vi "Do.vi"(8 "error in (no error)":errorcluster, 10 "Actor in":refnum<class "Actor.lvclass">, 11 "Get Indicators":refnum<class "Get Indicators.lvclass">) -> (0 "error out":errorcluster, 2 "Actor out":refnum<class "Actor.lvclass">)   [LabVIEW 2014, in "tWorkerCommandRunner.lvlib" / "Get Indicators.lvclass"]
doc: "(<B>Filename</B>: Actor Framework.lvlib:Message.lvclass:Do.vi)\n\nDefines what a message does when it is received by an actor. Generally, a message instructs an actor to invoke one of its methods. By default, this method does nothing. A child class must override it to define behavior. Create a child class by using the Actor Framework Message Maker dialog box."
uses:
  Get Indicators.lvclass
  <vilib>/ActorFramework/Actor/Actor.lvclass
  tWorkerCommandRunner/tWorkerCommandRunner.lvclass
  Get Indicators.lvclass/Get Indicators.ctl
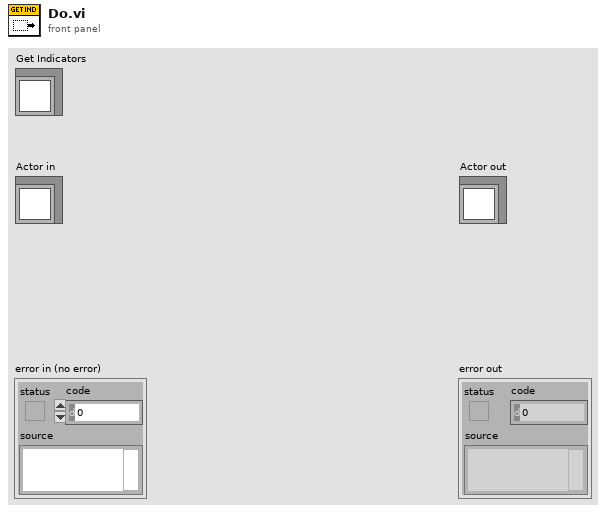
[diagram p1: front panel]
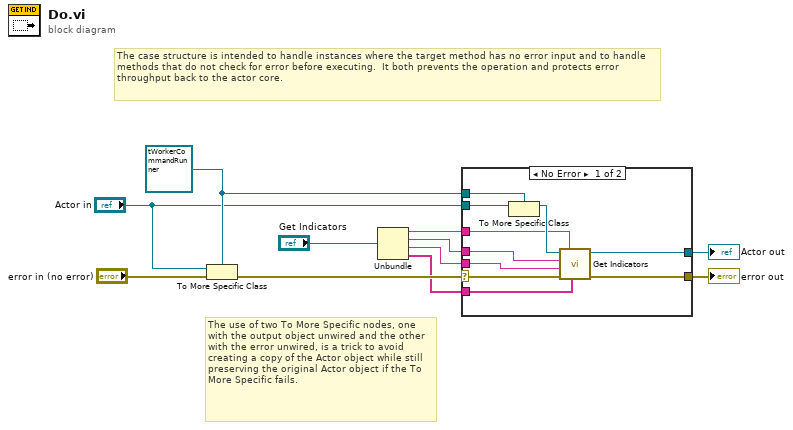
[diagram p0: block diagram]
diagram:
  w10 = refnum<class "tWorkerCommandRunner.lvclass"> refnum ("Actor in")
  # "The use of two To More Specific nodes, one with the output object unwired and the other with the error unwired, is a trick to avoid creating a copy of the Actor object while still preserving the original Actor object if the To More Specific fails."
  # "The case structure is intended to handle instances where the target method has no error input and to handle methods that do not check for error before executing.  It both prevents the operation and protects error throughput back to the actor core."
  n1 = To More Specific Class(target class=w10, reference="Actor in", error in="error in (no error)") -> (error out=w11:errorcluster)  [unwired: 1 out]
  n2 = Unbundle("Get Indicators") -> (w9:string, w8:string, w7:string, w6:string[])
  n3 = case shown="No Error" w11 {
    selector: w11 -> [w17 w23]
    tunnel: [w16 w23] -> w5
    tunnel: [w18 w22] -> w4
    tunnel: "Actor in" -> [w21 w22]
    tunnel: w10 -> [w20 _]
    tunnel: w9 -> [w14 _]
    tunnel: w8 -> [w13 _]
    tunnel: w7 -> [w12 _]
    tunnel: w6 -> [w15 _]
    frame No Error {
      n4 = To More Specific Class(target class=w20, reference=w21) -> (specific class reference=w19:refnum<class "tWorkerCommandRunner.lvclass">)  [unwired: 1 in, 1 out]
      n5 = call "Get Indicators.vi"("Control Names"=w15, "Project Path"=w14, "error in (no error)"=w17, "VI Path"=w12, "Target Name"=w13, "tWorkerCommandRunner in"=w19) -> ("error out"=w16:errorcluster, "tWorkerCommandRunner out"=w18:refnum<class "tWorkerCommandRunner.lvclass">)  [unwired: 4 in]
    }
    frame Error {
      # "If type check fails, pass the original object out again."
    }
  }
  "error out" <- w5
  "Actor out" <- w4
